vi "Helium Test - Step 2.vi"(7 "Step":i32, 8 "error in":errorcluster, 9 "Test Results In":T9, 10 "Gas":T8, 11 "Test Configuration":T1) -> (0 "error out":errorcluster, 1 "Test Results Out":T9, 2 "Gas Out":T8 caption="Gas", 3 "Test Configuration Out":T1)   [LabVIEW 2015]
uses:
  CAN Communication/PAS/Typedefs/Session Handle.ctl
  CAN Communication/PAS/PAS.lvclass
  Controls/Test Results.ctl
  Controls/Step Result.ctl
  Controls/Test Configuration.ctl
  Controls/Vacuum Test.ctl
  Controls/Test Timing.ctl
  Controls/Vaccum Thresholds.ctl
  Controls/Helium Test.ctl
  Controls/Helium Thresholds.ctl
  Controls/Functional Test.ctl
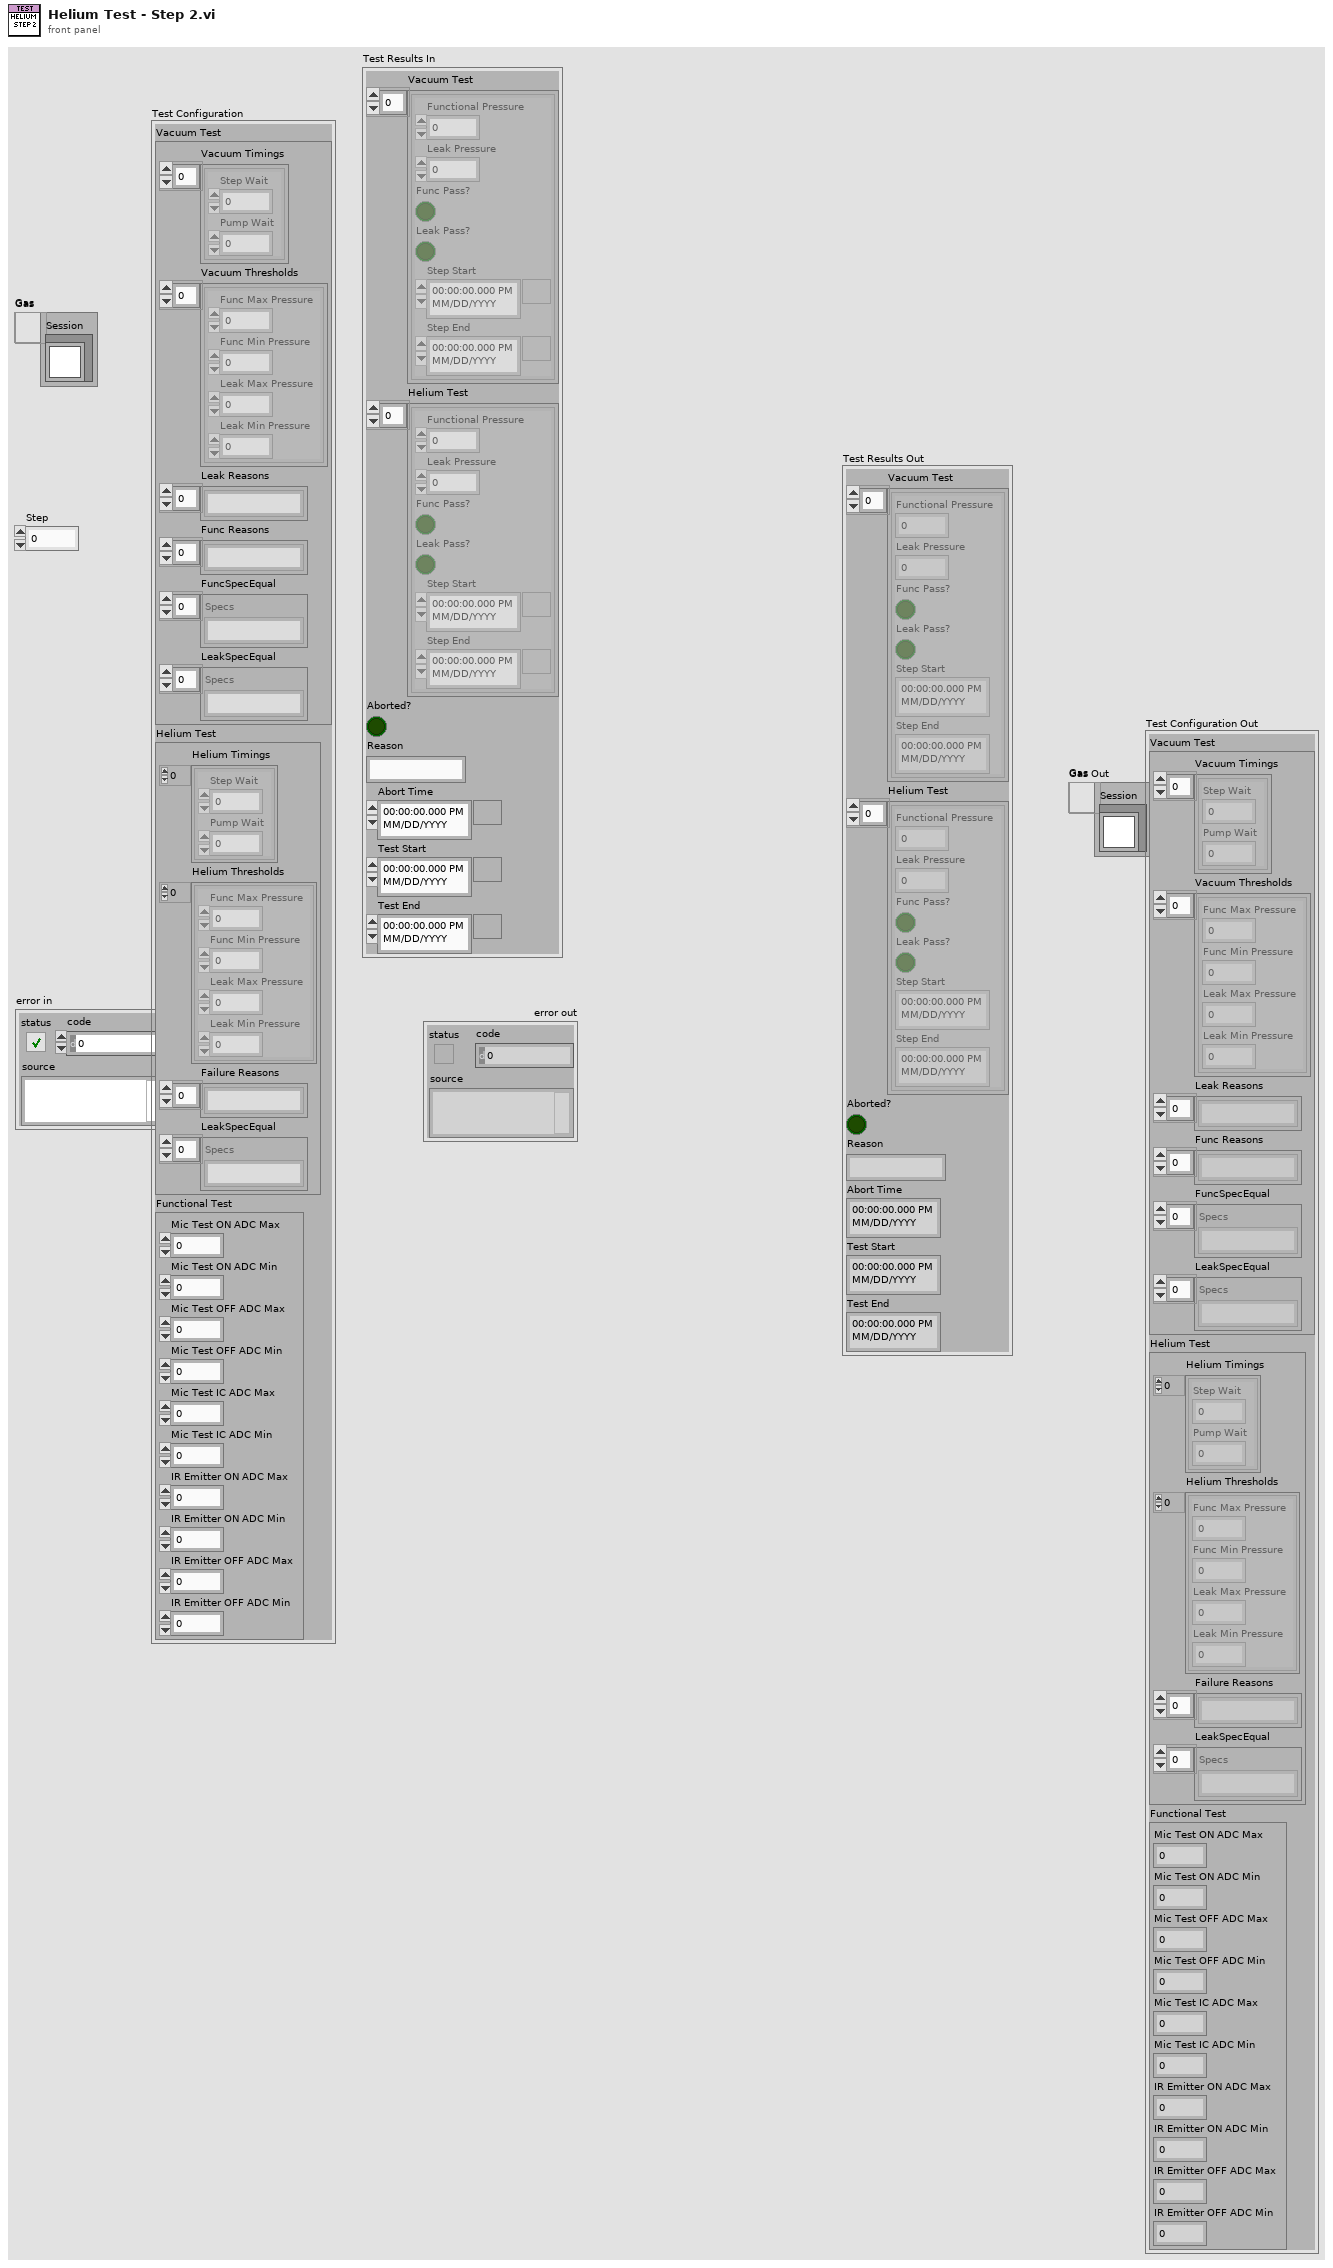
[diagram p1: front panel]
types:
  T1 = typedef "Test Configuration.ctl" = cluster{"Vacuum Test":T2, "Helium Test":T5, "Functional Test":T7}
  T2 = typedef "Vacuum Test.ctl" = cluster{"Vacuum Timings":T3[], "Vacuum Thresholds":T4[], "Leak Reasons":string[], "Func Reasons":string[], "FuncSpecEqual":string[], "LeakSpecEqual":string[]}
  T3 = typedef "Test Timing.ctl" = cluster{"Step Wait":dbl, "Pump Wait":dbl}
  T4 = typedef "Vaccum Thresholds.ctl" = cluster{"Func Max Pressure":dbl, "Func Min Pressure":dbl, "Leak Max Pressure":dbl, "Leak Min Pressure":dbl}
  T5 = typedef "Helium Test.ctl" = cluster{"Helium Timings":T3[], "Helium Thresholds":T6[], "Failure Reasons":string[], "LeakSpecEqual":string[]}
  T6 = typedef "Helium Thresholds.ctl" = cluster{"Func Max Pressure":dbl, "Func Min Pressure":dbl, "Leak Max Pressure":dbl, "Leak Min Pressure":dbl}
  T7 = typedef "Functional Test.ctl" = cluster{"Mic Test ON ADC Max":dbl, "Mic Test ON ADC Min":dbl, "Mic Test OFF ADC Max":dbl, "Mic Test OFF ADC Min":dbl, "Mic Test IC ADC Max":dbl, "Mic Test IC ADC Min":dbl, "IR Emitter ON ADC Max":dbl, "IR Emitter ON ADC Min":dbl, "IR Emitter OFF ADC Max":dbl, "IR Emitter OFF ADC Min":dbl}
  T8 = typedef "PAS.lvclass/Session Handle.ctl" = refnum<data-value>
  T9 = typedef "Test Results.ctl" = cluster{"Vacuum Test":T10[], "Helium Test":T10[], "Aborted?":bool, "Reason":string, "Abort Time":timestamp, "Test Start":timestamp, "Test End":timestamp}
  T10 = typedef "Step Result.ctl" = cluster{"Functional Pressure":dbl, "Leak Pressure":dbl, "Func Pass?":bool, "Leak Pass?":bool, "Step Start":timestamp, "Step End":timestamp}
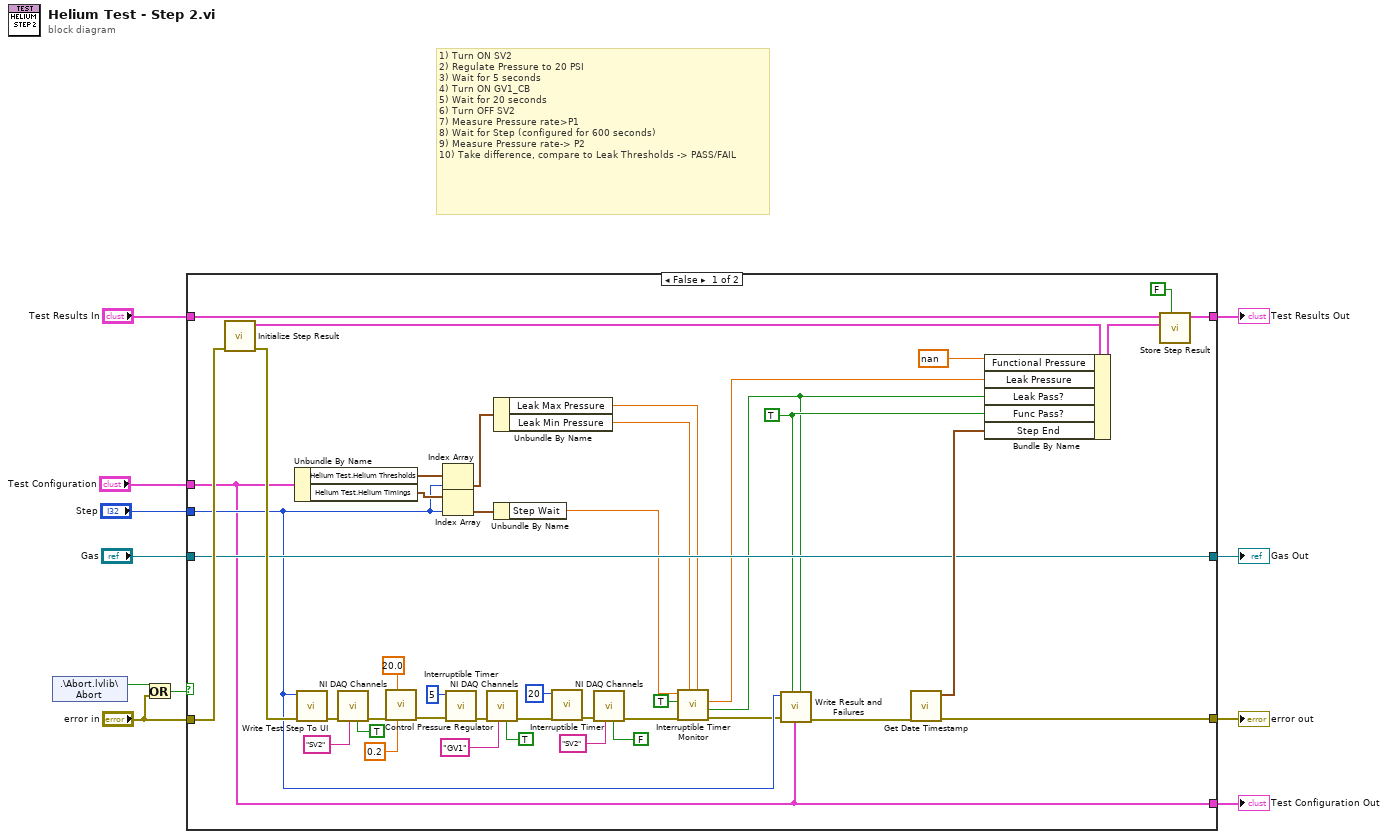
[diagram p0: block diagram]
diagram:
  # "1) Turn ON SV2\n2) Regulate Pressure to 20 PSI\n3) Wait for 5 seconds\n4) Turn ON GV1_CB\n5) Wait for 20 seconds\n6) Turn OFF SV2\n7) Measure Pressure rate>P1\n8) Wait for Step (configured for 600 seconds)\n9) Measure Pressure rate-> P2\n10) Take difference, compare to Leak Thresholds -> PASS/FAIL"
  n1 = shared-variable ".\\Abort.lvlib\\Abort"() -> (w10:bool)  [unwired: 1 in, 1 out]
  n2 = Or(x=w10, y="error in") -> (x .or. y?=w9:bool)
  n3 = case shown="False" w9 {
    tunnel: "error in" -> [w54 w57]
    tunnel: "Test Results In" -> [w51 w58]
    tunnel: [w52 w58] -> w7
    tunnel: [w15 w57] -> w6
    tunnel: "Test Configuration" -> [w41 w56]
    tunnel: "Step" -> [w42 _]
    tunnel: [w41 w56] -> w1
    tunnel: [w44 w55] -> w3
    tunnel: "Gas" -> [w44 w55]
    frame False {
      w39 = TRUE ("Func Pass?")
      n4 = call "Initialize Step Result.vi"("error in (no error)"=w54) -> ("error out"=w53:errorcluster, "New Step Result"=w50:T10)  [unwired: 8 in, 1 out]
      n5 = Unbundle By Name(w41) -> ("Helium Test.Helium Thresholds"=w47:T6[], "Helium Test.Helium Timings"=w46:T3[])
      n6 = call "Write Test Step To UI.vi"("error in (no error)"=w53, "Step"=w42) -> ("error out"=w33:errorcluster)  [unwired: 9 in]
      n7 = call "NI DAQ Channels.vi"("Control"=TRUE ("State"), "Channel"="SV2", "error in (no error)"=w33) -> ("error out"=w36:errorcluster)  [unwired: 7 in, 1 out]
      n8 = call "Control Pressure Regulator.vi"("y"=0.2, "error in"=w36, "Desired PSI"=20.0) -> ("error out"=w34:errorcluster)  [unwired: 7 in, 1 out]
      n9 = Index Array(array=w47, index=w42) -> (element=w43:T6)
      n10 = Index Array(array=w46, index=w42) -> (element=w45:T3)
      n11 = call "Interruptible Timer.vi"("error in (no error)"=w34, "Wait (s)"=5) -> ("error out"=w32:errorcluster)  [unwired: 7 in, 2 out]
      n12 = call "NI DAQ Channels.vi"("Control"=TRUE ("State"), "Channel"="GV1", "error in (no error)"=w32) -> ("error out"=w29:errorcluster)  [unwired: 7 in, 1 out]
      n13 = Unbundle By Name(w43) -> ("Leak Max Pressure"=w22:dbl, "Leak Min Pressure"=w23:dbl)
      n14 = Unbundle By Name(w45) -> ("Step Wait"=w25:dbl)
      n15 = call "Interruptible Timer.vi"("error in (no error)"=w29, "Wait (s)"=20) -> ("error out"=w28:errorcluster)  [unwired: 7 in, 2 out]
      n16 = call "NI DAQ Channels.vi"("Control"=FALSE ("State"), "Channel"="SV2", "error in (no error)"=w28) -> ("error out"=w26:errorcluster)  [unwired: 7 in, 1 out]
      n17 = call "Interruptible Timer Monitor.vi"("Max"=w22, "Min"=w23, "error in (no error)"=w26, "Update UI?"=TRUE, "Wait (s)"=w25) -> ("error out"=w17:errorcluster, "In Range?"=w20:bool, "Leak Rate"=w21:dbl)  [unwired: 2 in, 2 out]
      n18 = call "Write Result and Failures.vi"("Leak"=w20, "Test Configuration"=w41, "Func"=w39, "error in (no error)"=w17, "Step"=w42) -> ("error out"=w16:errorcluster)  [unwired: 6 in]
      n19 = call "Get Date Timestamp.vi"("error in (no error)"=w16) -> ("error out"=w15:errorcluster, "current time"=w48:timestamp)  [unwired: 9 in]
      n20 = Bundle By Name(cluster=w50, "Functional Pressure"=nan, "Leak Pressure"=w21, "Leak Pass?"=w20, "Func Pass?"=w39, "Step End"=w48) -> (w49:T10)
      n21 = call "Store Step Result.vi"("Vacuum?"=FALSE, "Step Result"=w49, "Test Results In"=w51) -> ("Test Results Out"=w52:T9)  [unwired: 8 in]
    }
    frame True {
    }
  }
  "error out" <- w6
  "Test Results Out" <- w7
  "Gas Out" <- w3
  "Test Configuration Out" <- w1
